vi "Shooter_WinchNoPID.vi"(8 "Winch Pot Location":dbl, 9 "fired":dbl, 10 "Buttons":T1, 11 "SetPointArray":dbl[](array[numeric])=[1.0, 2.0, 3.0]) -> (3 "Winch Motor Power Out":dbl)   [LabVIEW 2013]
uses:
  <vilib>/Rock Robotics/WPI/Joystick/WPI_JoystickButtonState.ctl
panel:
  in  "WinchPower":dbl=0.75
  out "Winch Desired Location":dbl
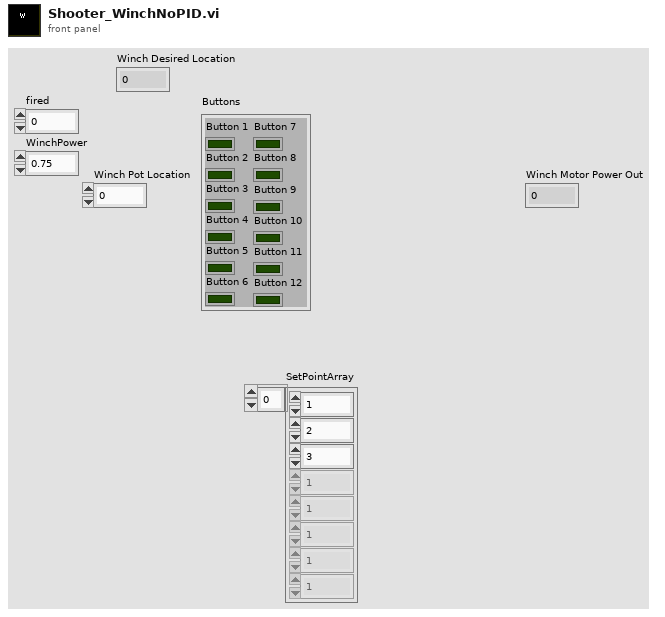
[diagram p1: front panel]
types:
  T1 = typedef "WPI_JoystickButtonState.ctl" = cluster{"Button 1":bool, "Button 2":bool, "Button 3":bool, "Button 4":bool, "Button 5":bool, "Button 6":bool, "Button 7":bool, "Button 8":bool, "Button 9":bool, "Button 10":bool, "Button 11":bool, "Button 12":bool}
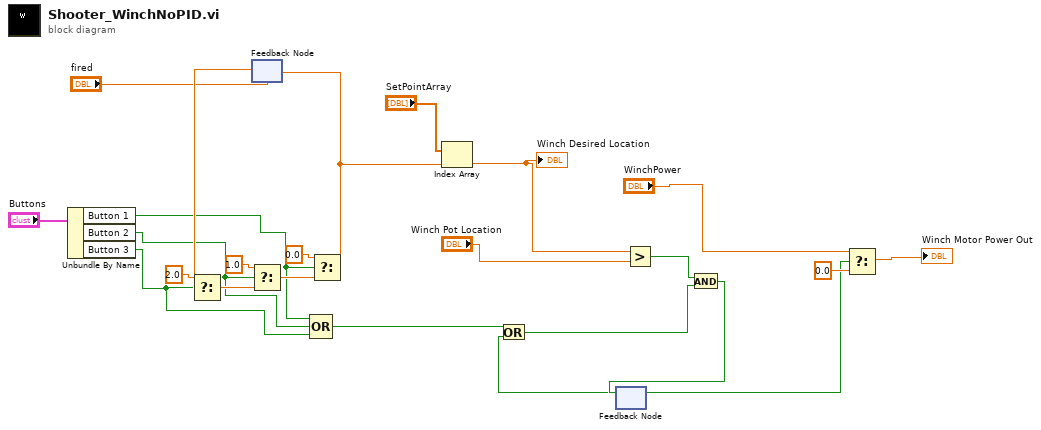
[diagram p0: block diagram]
diagram:
  n1 = Unbundle By Name("Buttons") -> ("Button 1"=w11:bool, "Button 2"=w12:bool, "Button 3"=w13:bool)
  n2 = feedback #1("fired") -> (w17:dbl)
  n3 = Select(t=2.0, s=w13, f=w17) -> (s? t:f=w23:dbl)
  n4 = Select(t=1.0, s=w12, f=w23) -> (s? t:f=w22:dbl)
  n5 = Compound Arithmetic op=OR(w11, w12, w13) -> (w16:bool)
  n6 = Select(t=0.0, s=w11, f=w22) -> (s? t:f=w15:dbl)
  n7 = feedback-in #1(w15) -> ()
  n8 = Index Array(array="SetPointArray", index=w15) -> (element=w9:dbl)
  "Winch Desired Location" <- w9
  n9 = feedback #2() -> (w2:bool)  [unwired: 1 in]
  n10 = Or(x=w16, y=w2) -> (x .or. y?=w5:bool)
  n11 = Greater?(x=w9, y="Winch Pot Location") -> (0:w4:bool)
  n12 = And(x=w4, y=w5) -> (x .and. y?=w3:bool)
  n13 = feedback-in #2(w3) -> ()
  n14 = Select(t="WinchPower", s=w2, f=0.0) -> (s? t:f=→"Winch Motor Power Out":dbl)
